vi "Pruebas y tareas.vi"() -> ()   [LabVIEW 2019]
uses:
  <vilib>/Instr/_visa.llb/VISA Configure Serial Port (Instr).vi
panel:
  out "String":string
  out "Numeric":i32
  out "Gauge":dbl(knob) scale=0.0..10.0
  out "Thermometer":i32(slide) scale=0.0..100.0
  in  "WRITE":bool
  in  "write buffer":string
  in  "stop":bool
  out "read buffer":string
  in  "VISA resource name 2":refnum<visa-resource-name>
  in  "READ":bool
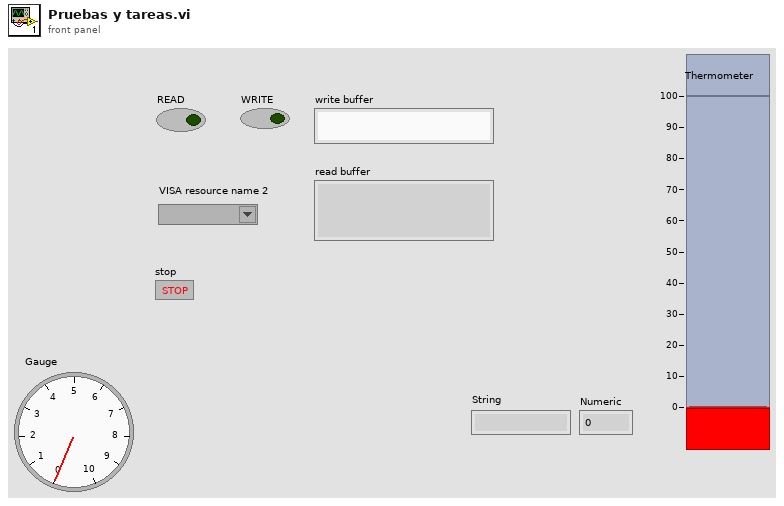
[diagram p1: front panel]
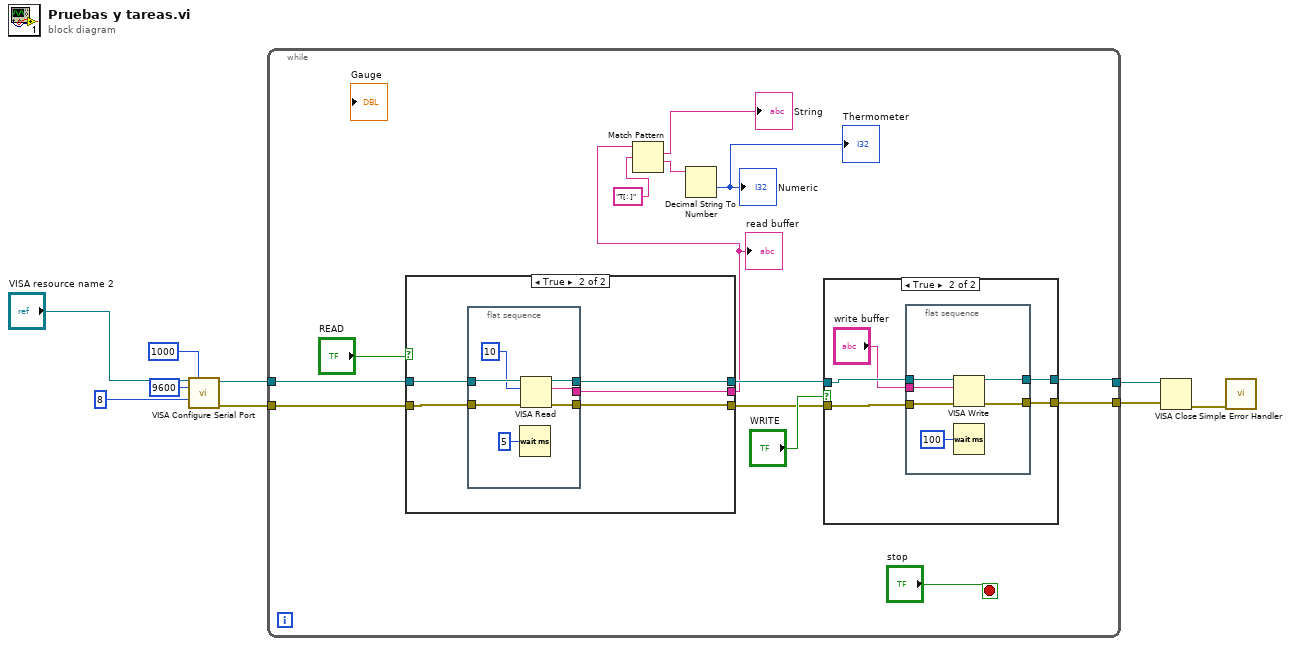
[diagram p0: block diagram]
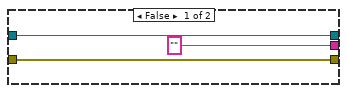
[diagram p3: hidden frame]
diagram:
  n1 = call-poly "VISA Configure Serial Port"("VISA resource name"="VISA resource name 2", "timeout (10sec)"=u32 1000, "baud rate (9600)"=u32 9600, "data bits (8)"=u16 8) -> ("VISA resource name out"=w8:refnum<visa-resource-name>, "error out"=w7:errorcluster)  [unwired: 5 in, 5 out]
  n2 = while {
    tunnel: w8 -> [w21]
    tunnel: w7 -> [w19]
    tunnel: [w16] -> w3
    tunnel: [w15] -> w2
    stop <- "stop" stop-if-true
    n3 = case shown="True" "READ" {
      tunnel: w21 -> [w39 w44]
      tunnel: w19 -> [w38 w43]
      tunnel: [w39 w41] -> w18
      tunnel: [w38 w42] -> w17
      tunnel: ["" ("read buffer") w40] -> w10
      frame False {
      }
      frame True {
        n4 = flat-sequence {
          tunnel: w44 -> [w51]
          tunnel: w43 -> [w50]
          tunnel: [w49] -> w41
          tunnel: [w48] -> w42
          tunnel: [w47] -> w40
          frame #0 {
            n5 = Wait (ms)(milliseconds to wait=u32 5) -> ()  [unwired: 1 out]
            n6 = VISA Read(VISA resource name=w51, byte count=u32 10, error in (no error)=w50) -> (VISA resource name out=w49:refnum<visa-resource-name>, read buffer=w47:string, error out=w48:errorcluster)  [unwired: 1 out]
          }
        }
      }
    }
    "read buffer" <- w10
    n7 = Match Pattern(string=w10, regular expression="T[: ]") -> (match substring=→"String":string, after substring=w14:string)  [unwired: 1 in, 2 out]
    n8 = Decimal String To Number(string=w14) -> (number=→"Thermometer" →"Numeric":i32)  [unwired: 2 in, 1 out]
    n9 = case shown="True" "WRITE" {
      tunnel: w18 -> [w25 w30]
      tunnel: w17 -> [w24 w29]
      tunnel: [w25 w27] -> w16
      tunnel: [w24 w26] -> w15
      frame False {
      }
      frame True {
        n10 = flat-sequence {
          tunnel: w30 -> [w36]
          tunnel: w29 -> [w35]
          tunnel: "write buffer" -> [w34]
          tunnel: [w33] -> w27
          tunnel: [w32] -> w26
          frame #0 {
            n11 = VISA Write(VISA resource name=w36, write buffer=w34, error in (no error)=w35) -> (VISA resource name out=w33:refnum<visa-resource-name>, error out=w32:errorcluster)  [unwired: 1 out]
            n12 = Wait (ms)(milliseconds to wait=u32 100) -> ()  [unwired: 1 out]
          }
        }
      }
    }
  }
  n13 = VISA Close(VISA resource name=w3, error in (no error)=w2) -> (error out=w9:errorcluster)
  n14 = call <vilib>:"Simple Error Handler.vi"("error in (no error)"=w9) -> ()  [unwired: 1 in, 8 out]
